vi "verify-selected-wavesSD.vi"(0 "in wave":dbl format="%#_13g", 1 "selected wavelengths":dbl[](array[numeric])=[550.0, 640.0, 680.0, 720.0, 780.0, 800.0]) -> (2 "closet wave":dbl, 3 "closest index":i32, 4 "selected wavelengths out":dbl[](array[numeric])=[550.0, 640.0, 680.0, 720.0, 780.0, 800.0], 5 "closet indexes":i32[](array[numeric]))   [LabVIEW 2015]
uses:
  globalVarSD.vi
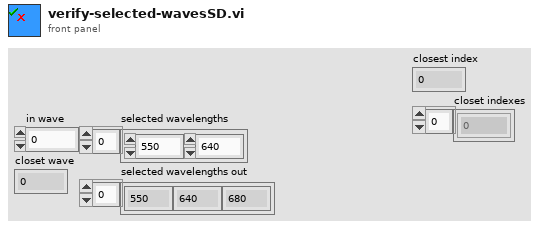
[diagram p1: front panel]
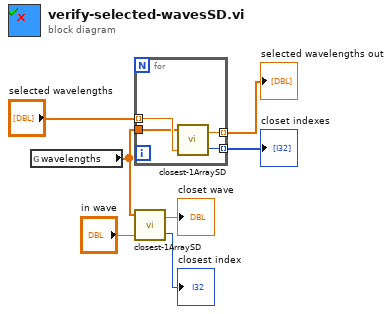
[diagram p0: block diagram]
diagram:
  n1 = global read "globalVarSD.vi" "wavelengths"() -> (w5:dbl[])
  n2 = for {
    tunnel: "selected wavelengths" -> [w11] mode=indexing
    tunnel: w5 -> [w10]
    tunnel: [w9] -> w6 mode=indexing
    tunnel: [w8] -> w1 mode=indexing
    n3 = call "closest-1ArraySD.vi"("desired element"=w11, "1D Array"=w10) -> ("closest index"=w8:i32, "closest element"=w9:dbl)  [unwired: 1 in]
  }
  "selected wavelengths out" <- w6
  "closet indexes" <- w1
  n4 = call "closest-1ArraySD.vi"("desired element"="in wave", "1D Array"=w5) -> ("closest index"=→"closest index":i32, "closest element"=→"closet wave":dbl)  [unwired: 1 in]
